vi "FormLogin-.vi"() -> ()   [LabVIEW 2013]
uses:
  <vilib>/addons/database/_DB Variant To Data/Database Variant To Data.xnode
panel:
  out "管理员":string(combo)
  out "编号":string(combo)
  in  "联机模式":enum32{"未选择", "联网模式", "单机模式"}(radio)
  in  "用户登录":bool
  out "udl名称":string="epsacc.udl"
  in  "修改密码":bool
  in  "用户名":string(combo)
  in  "密码":string
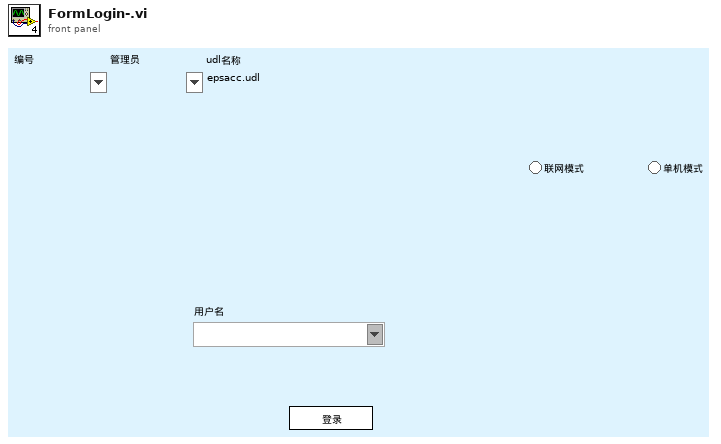
[diagram p1: front panel]
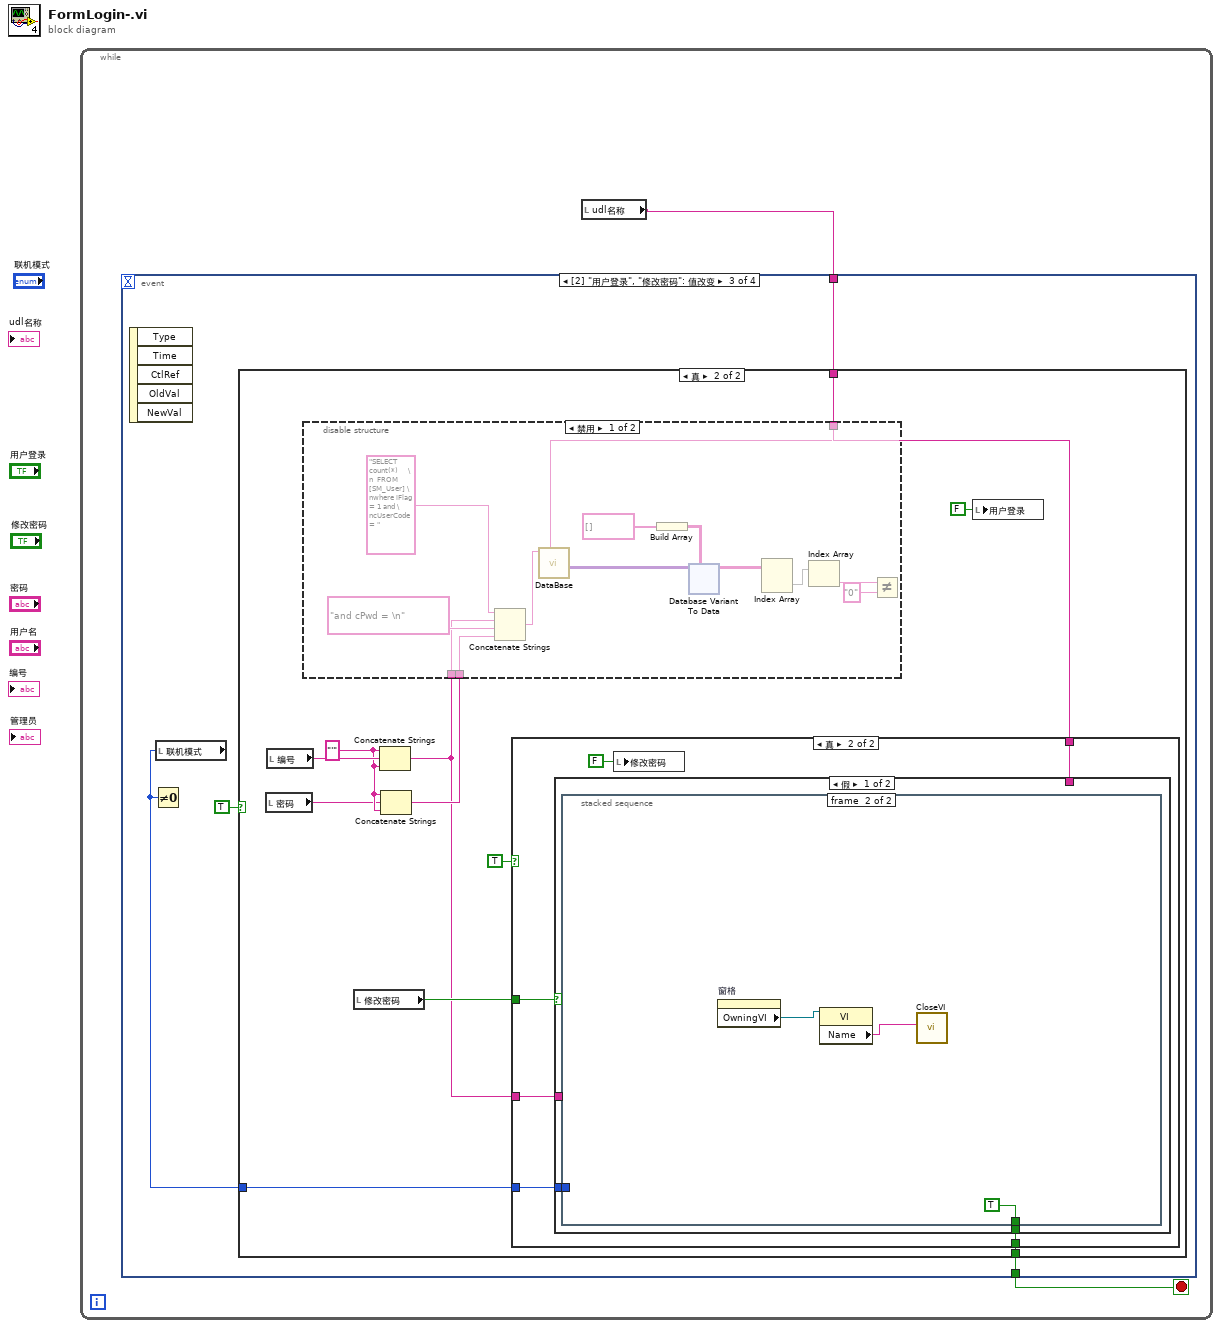
[diagram p0: block diagram]
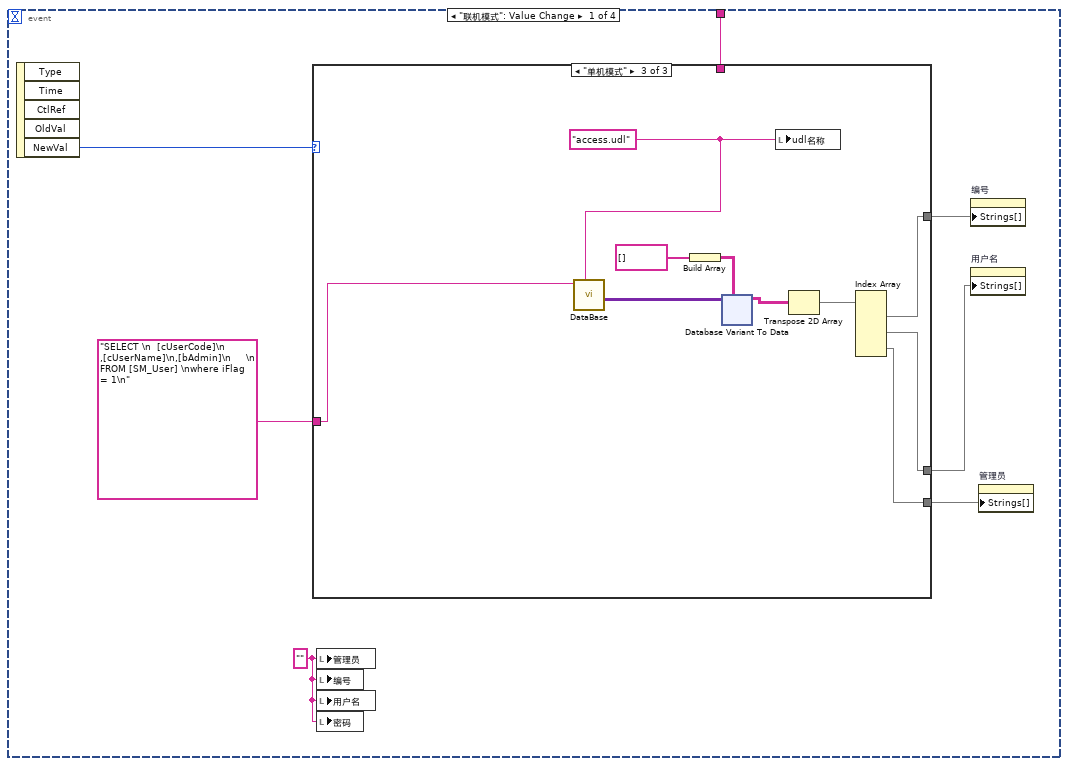
[diagram p2: hidden frame]
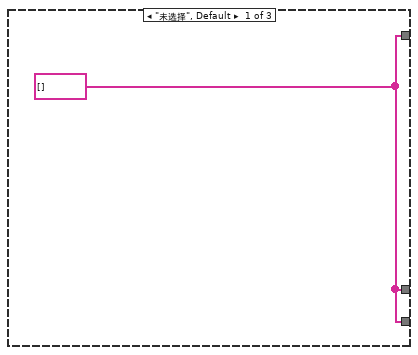
[diagram p3: hidden frame]
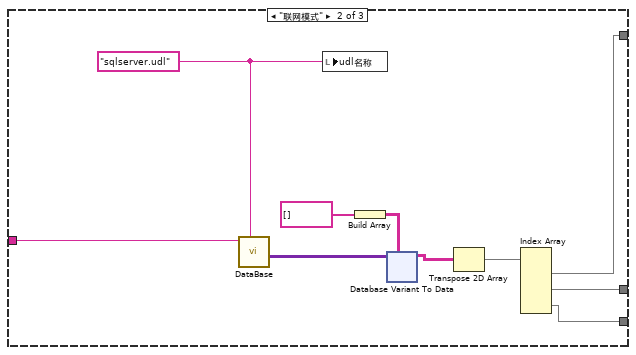
[diagram p4: hidden frame]
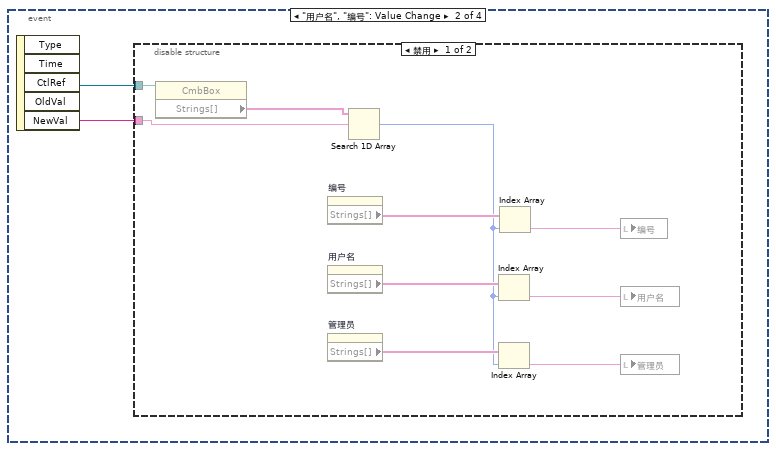
[diagram p5: hidden frame]
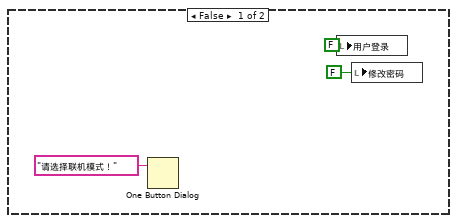
[diagram p7: hidden frame]
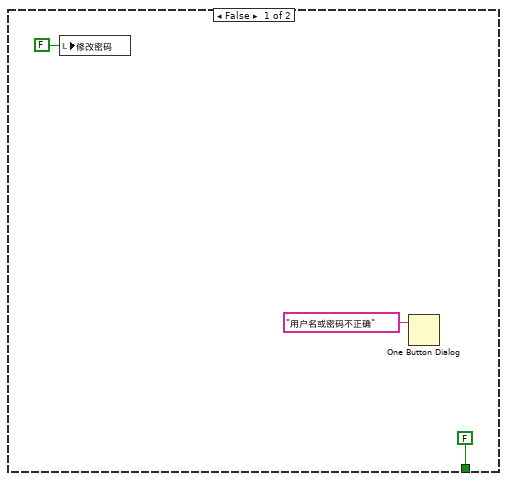
[diagram p9: hidden frame]
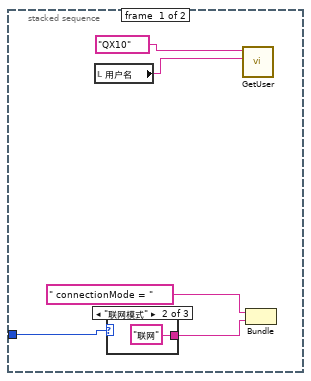
[diagram p10: hidden frame]
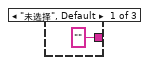
[diagram p11: hidden frame]
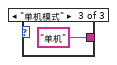
[diagram p12: hidden frame]
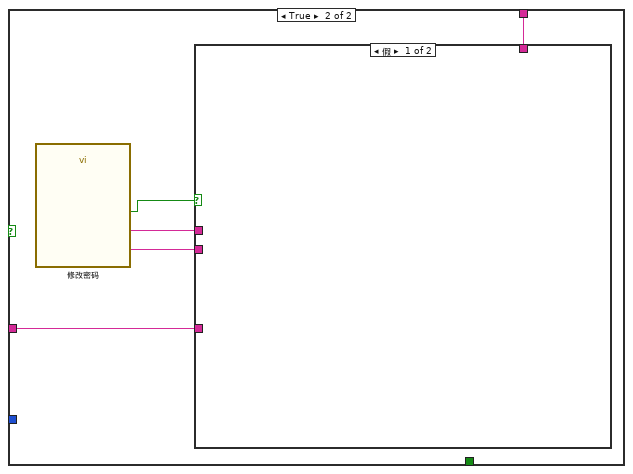
[diagram p13: hidden frame]
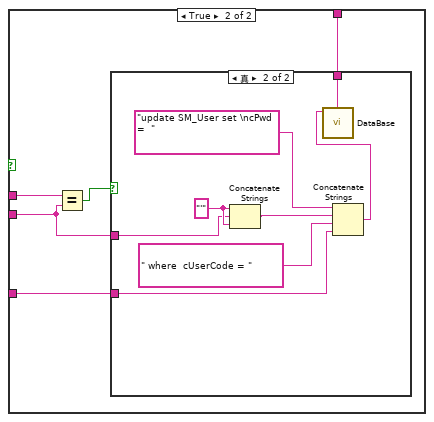
[diagram p14: hidden frame]
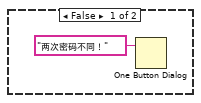
[diagram p15: hidden frame]
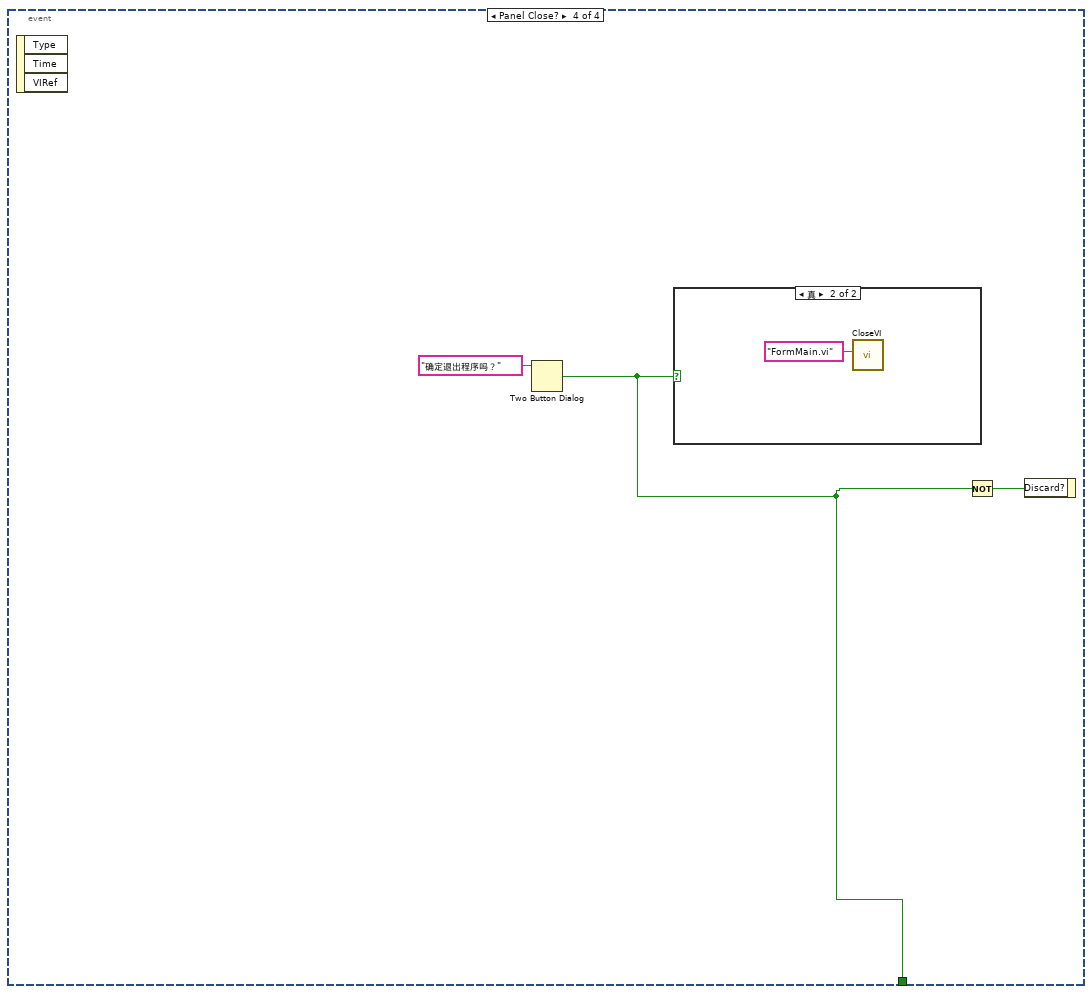
[diagram p16: hidden frame]
diagram:
  n1 = while {
    stop <- w2 stop-if-true
    n2 = local read "udl名称"() -> (w1:string)
    n3 = event shown="[2] \"用户登录\", \"修改密码\": 值改变" {
      selector: _ -> [_ _ _ _]
      dyn-events: _ -> [_ _ _ _]
      timeout: _ -> [_ _ _ _]
      tunnel: [_ _ w134 w247] -> w2
      tunnel: w1 -> [w8 _ w133 _]
      event "联机模式": Value Change {
        w3 = "" ("密码")
        n4 = event-data() -> ("NewVal"=w9:enum32{"未选择", "联网模式", "单机模式"})  [unwired: 1 in, 4 out]
        n5 = case shown="\"单机模式\"" w9 {
          tunnel: w8 -> [_ _ _]
          tunnel: [w10 w14 w69] -> w7
          tunnel: "SELECT \n  [cUserCode]\n     ,[cUserName]\n,[bAdmin]\n     \n  FROM [SM_User] \nwhere iFlag = 1\n" ("SQL query") -> [_ w13 w67]
          tunnel: [w10 w12 w66] -> w5
          tunnel: [w10 w11 w65] -> w4
          frame "未选择", Default {
            w10 = string[] [] ("字符串[]")
          }
          frame "联网模式" {
            w15 = "sqlserver.udl" ("udl名称")
            n6 = call "DataBase.vi"("udl名称"=w15, "SQL query"=w13) -> ("recordset data"=w17:variant[][])  [unwired: 9 in]
            n7 = local write "udl名称"(w15) -> ()
            n8 = Build Array(string[] [] ("添加的数组")) -> (w19:string[][])
            n9 = xnode "Database Variant To Data"("database variant"=w17, "type"=w19) -> ("data"=w18:string[][])  [unwired: 1 in, 1 out]
            n10 = Transpose 2D Array(2D array=w18) -> (transposed array=w16:string[][])
            n11 = Index Array(array=w16) -> (element #1=w14:string[], element #2=w12:string[], element #3=w11:string[])  [unwired: 6 in]
          }
          frame "单机模式" {
            w68 = "access.udl" ("udl名称")
            n12 = call "DataBase.vi"("udl名称"=w68, "SQL query"=w67) -> ("recordset data"=w71:variant[][])  [unwired: 9 in]
            n13 = Build Array(string[] [] ("添加的数组")) -> (w73:string[][])
            n14 = xnode "Database Variant To Data"("database variant"=w71, "type"=w73) -> ("data"=w72:string[][])  [unwired: 1 in, 1 out]
            n15 = local write "udl名称"(w68) -> ()
            n16 = Transpose 2D Array(2D array=w72) -> (transposed array=w70:string[][])
            n17 = Index Array(array=w70) -> (element #1=w69:string[], element #2=w66:string[], element #3=w65:string[])  [unwired: 6 in]
          }
        }
        n18 = local write "管理员"(w3) -> ()
        n19 = local write "编号"(w3) -> ()
        n20 = local write "用户名"(w3) -> ()
        n21 = local write "密码"(w3) -> ()
        n22 = property on="编号" class="CmbBox"("Strings[]"=w7) -> ()  [unwired: 2 in, 2 out]
        n23 = property on="用户名" class="CmbBox"("Strings[]"=w5) -> ()  [unwired: 2 in, 2 out]
        n24 = property on="管理员" class="CmbBox"("Strings[]"=w4) -> ()  [unwired: 2 in, 2 out]
      }
      event "用户名", "编号": Value Change {
        n25 = event-data() -> ("CtlRef"=w120:refnum<vi>, "NewVal"=w119:string)  [unwired: 1 in, 3 out]
        n26 = disable-structure shown="禁用" {
          disable-tunnel: w120 -> [w130 _]
          disable-tunnel: w119 -> [w128 _]
          frame Disabled {
            n27 = property class="CmbBox"(reference=w130) -> ("Strings[]"=w129:string[])  [unwired: 1 in, 2 out]
            n28 = property on="编号" class="CmbBox"() -> ("Strings[]"=w127:string[])  [unwired: 2 in, 2 out]
            n29 = property on="用户名" class="CmbBox"() -> ("Strings[]"=w126:string[])  [unwired: 2 in, 2 out]
            n30 = property on="管理员" class="CmbBox"() -> ("Strings[]"=w122:string[])  [unwired: 2 in, 2 out]
            n31 = Search 1D Array(1D array=w129, element=w128) -> (index of element=w121:i32)  [unwired: 1 in]
            n32 = Index Array(array=w126, index=w121) -> (element=w124:string)
            n33 = Index Array(array=w122, index=w121) -> (element=w123:string)
            n34 = Index Array(array=w127, index=w121) -> (element=w125:string)
            n35 = local write "编号"(w125) -> ()
            n36 = local write "用户名"(w124) -> ()
            n37 = local write "管理员"(w123) -> ()
          }
          frame Enabled {
          }
        }
      }
      event "用户登录", "修改密码": Value Change {
        n38 = event-data() -> ()  [unwired: 1 in, 5 out]
        n39 = local read "联机模式"() -> (w132:enum32{"未选择", "联网模式", "单机模式"})
        n40 = Not Equal To 0?(x=w132) -> ()  [unwired: 1 out]
        n41 = case shown="真" TRUE {
          tunnel: [_ w148] -> w134
          tunnel: w133 -> [_ w139]
          tunnel: w132 -> [_ w141]
          frame False {
            n42 = One Button Dialog(message="请选择联机模式！" ("消息")) -> ()  [unwired: 1 in, 1 out]
            n43 = local write "用户登录"(FALSE ("登录")) -> ()
            n44 = local write "修改密码"(FALSE ("登录")) -> ()
          }
          frame True {
            w146 = "'"
            n45 = local read "密码"() -> (w145:string)
            n46 = local read "编号"() -> (w147:string)
            n47 = local read "修改密码"() -> (w143:bool)
            n48 = Concatenate Strings(w146, w147, w146) -> (w140:string)
            n49 = Concatenate Strings(w146, w145, w146) -> (w144:string)
            n50 = disable-structure shown="禁用" {
              disable-tunnel: w144 -> [w156 _]
              disable-tunnel: w140 -> [w150 _]
              disable-tunnel: w139 -> [w149 _]
              frame Disabled {
                n51 = Concatenate Strings("SELECT count(*)     \n  FROM [SM_User] \nwhere iFlag = 1 and \ncUserCode = " ("SQL query"), w150, "and cPwd = \n" ("SQL query"), w156) -> (w155:string)
                n52 = call "DataBase.vi"("udl名称"=w149, "SQL query"=w155) -> ("recordset data"=w159:variant[][])  [unwired: 9 in]
                n53 = Build Array(string[] [] ("添加的数组")) -> (w160:string[][])
                n54 = xnode "Database Variant To Data"("database variant"=w159, "type"=w160) -> ("data"=w154:string[][])  [unwired: 1 in, 1 out]
                n55 = Index Array(array=w154) -> (element=w153:string[])  [unwired: 2 in]
                n56 = Index Array(array=w153) -> (element=w152:string)  [unwired: 1 in]
                n57 = Not Equal?(x=w152, y="0") -> ()  [unwired: 1 out]
              }
              frame Enabled {
              }
            }
            n58 = case shown="真" TRUE {
              tunnel: [FALSE w214] -> w148
              tunnel: w143 -> [_ w213]
              tunnel: w141 -> [_ w211]
              tunnel: w140 -> [_ w210]
              tunnel: w139 -> [_ w209]
              frame False {
                n59 = local write "修改密码"(FALSE ("登录")) -> ()
                n60 = One Button Dialog(message="用户名或密码不正确" ("消息")) -> ()  [unwired: 1 in, 1 out]
              }
              frame True {
                n61 = case shown="假" w213 {
                  tunnel: [w216 _] -> w214
                  tunnel: w211 -> [w215 _]
                  tunnel: w210 -> [_ w229]
                  tunnel: w209 -> [_ w228]
                  frame False {
                    n62 = stacked-sequence {
                      tunnel: [_ TRUE] -> w216
                      tunnel: w215 -> [w221 _]
                      frame #0 {
                        n63 = local read "用户名"() -> (w217:string)
                        n64 = case shown="\"联网模式\"" w221 {
                          tunnel: ["" "联网" "单机"] -> w220
                          frame "未选择", Default {
                          }
                          frame "联网模式" {
                          }
                          frame "单机模式" {
                          }
                        }
                        n65 = call "GetUser.vi"("string"=w217, "权限"="QX10") -> ()  [unwired: 7 in, 3 out]
                        n66 = Bundle("y"=" connectionMode = ", w220) -> ()  [unwired: 1 in, 1 out]
                      }
                      frame #1 {
                        n67 = property on="窗格" class="Pane"() -> ("OwningVI"=w226:refnum<vi>)  [unwired: 2 in, 2 out]
                        n68 = property class="VI"(reference=w226) -> ("Name"=w225:string)  [unwired: 1 in, 2 out]
                        n69 = call "CloseVI.vi"("名称或相对路径"=w225) -> ()  [unwired: 10 in, 1 out]
                      }
                    }
                  }
                  frame True {
                    n70 = call "修改密码"() -> ("确认密码"=w230:string, "新密码"=w231:string, "确定"=w232:bool)  [unwired: 16 in, 1 out]
                    n71 = case shown="假" w232 {
                      tunnel: w231 -> [_ w237]
                      tunnel: w230 -> [_ w234]
                      tunnel: w228 -> [_ w235]
                      tunnel: w229 -> [_ w233]
                      frame False {
                      }
                      frame True {
                        n72 = Equal?(x=w237, y=w234) -> (x = y?=w236:bool)
                        n73 = case shown="真" w236 {
                          tunnel: w235 -> [_ w246]
                          tunnel: w234 -> [_ w239]
                          tunnel: w233 -> [_ w243]
                          frame False {
                            n74 = One Button Dialog(message="两次密码不同！" ("消息")) -> ()  [unwired: 1 in, 1 out]
                          }
                          frame True {
                            w241 = "'"
                            n75 = Concatenate Strings(w241, w239, w241) -> (w240:string)
                            n76 = Concatenate Strings("update SM_User set \ncPwd =  " ("SQL query"), w240, " where  cUserCode = " ("SQL query"), w243) -> (w242:string)
                            n77 = call "DataBase.vi"("udl名称"=w246, "SQL query"=w242) -> ()  [unwired: 9 in, 1 out]
                          }
                        }
                      }
                    }
                  }
                }
                n78 = local write "修改密码"(FALSE ("登录")) -> ()
              }
            }
            n79 = local write "用户登录"(FALSE ("登录")) -> ()
          }
        }
      }
      event Panel Close? {
        n80 = event-data() -> ()  [unwired: 1 in, 3 out]
        n81 = Two Button Dialog(message="确定退出程序吗？" ("消息")) -> (T button?=w247:bool)  [unwired: 2 in]
        n82 = case shown="真" w247 {
          frame False {
          }
          frame True {
            n83 = call "CloseVI.vi"("名称或相对路径"="FormMain.vi") -> ()  [unwired: 10 in, 1 out]
          }
        }
        n84 = Not(x=w247) -> (.not. x?=w248:bool)
        n85 = event-data("Discard?"=w248) -> ()  [unwired: 1 in, 1 out]
      }
    }
  }
